vi "Add.vi"(8 "Y":dbl, 11 "X":dbl) -> (3 "X+Y":dbl)   [LabVIEW 2019, in "Siple Math Toolkit.lvlib"]
uses:
  Siple Math Toolkit.lvlib
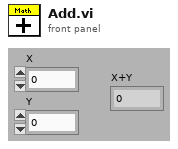
[diagram p1: front panel]
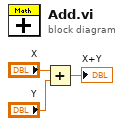
[diagram p0: block diagram]
diagram:
  n1 = Add(x="X", y="Y") -> (x+y=→"X+Y":dbl)
